vi "readoutport.vi"() -> ()   [LabVIEW 2010]
panel:
  in  "Readout port":u32
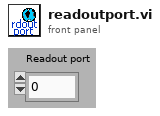
[diagram p1: front panel]
diagram:
